vi "set_intensity_modifier.vi"(8 "error in (no error)":errorcluster, 10 "intensity modifier":refnum<class "GenericAnalogOut.lvclass">, 11 "ScanHeadMH100729FPGA in":refnum<class "ScanHeadMH100729FPGA.lvclass">) -> (0 "error out":errorcluster, 3 "ScanHeadMH100729FPGA out":refnum<class "ScanHeadMH100729FPGA.lvclass">)   [LabVIEW 2010, in "ScanHeadMH100729FPGA.lvclass"]
uses:
  ScanHeadMH100729FPGA.lvclass
  AnalogOut/GenericAnalogOut/GenericAnalogOut/GenericAnalogOut.lvclass
  ScanHeadMH100729FPGA.lvclass/ScanHeadMH100729FPGA.ctl
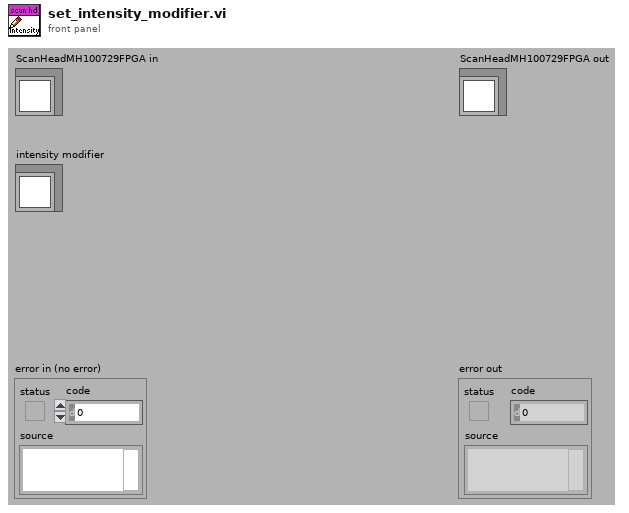
[diagram p1: front panel]
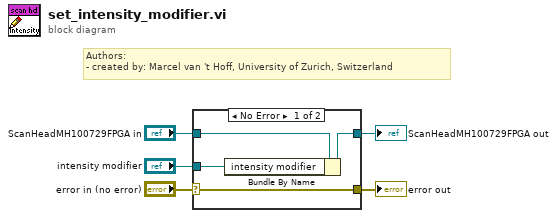
[diagram p0: block diagram]
diagram:
  # "Authors: \n- created by: Marcel van 't Hoff, University of Zurich, Switzerland"
  n1 = case shown="No Error" "error in (no error)" {
    selector: "error in (no error)" -> [w9 w11]
    tunnel: [w9 w11] -> w4
    tunnel: [w7 w10] -> w2
    tunnel: "ScanHeadMH100729FPGA in" -> [w8 w10]
    tunnel: "intensity modifier" -> [w6 _]
    frame No Error {
      n2 = Bundle By Name(cluster=w8, "intensity modifier"=w6) -> (w7:refnum<class "ScanHeadMH100729FPGA.lvclass">)
    }
    frame Error {
    }
  }
  "error out" <- w4
  "ScanHeadMH100729FPGA out" <- w2
